vi "3 Balls.vi"() -> ()   [LabVIEW 2019]
uses:
  Team Code/TurretMode.ctl
  Team Code/MotorsGlobal.vi
  Team Code/JoysticksGlobal.vi
  Default3BallEnum.ctl
panel:
  in  "TimeLimit_Atira":dbl
  in  "3BallPID":enum32{"AndaAtras1", "AlinhaLL"}(tab)
  in  "DistanceAtras1":dbl
  in  "DelayAndaAtras1":i32=300
  in  "TimeLimit_AlinhaLL":dbl
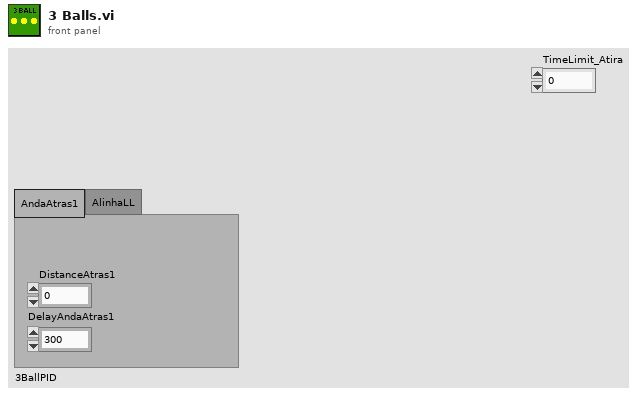
[diagram p1: front panel]
types:
  T1 = typedef "TurretMode.ctl" = enum16{"Static", "Manual", "Automatic"}
  T2 = typedef "Default3BallEnum.ctl" = enum16{"Reset1", "AndaAtras1", "AlinhaLL", "Atira"}
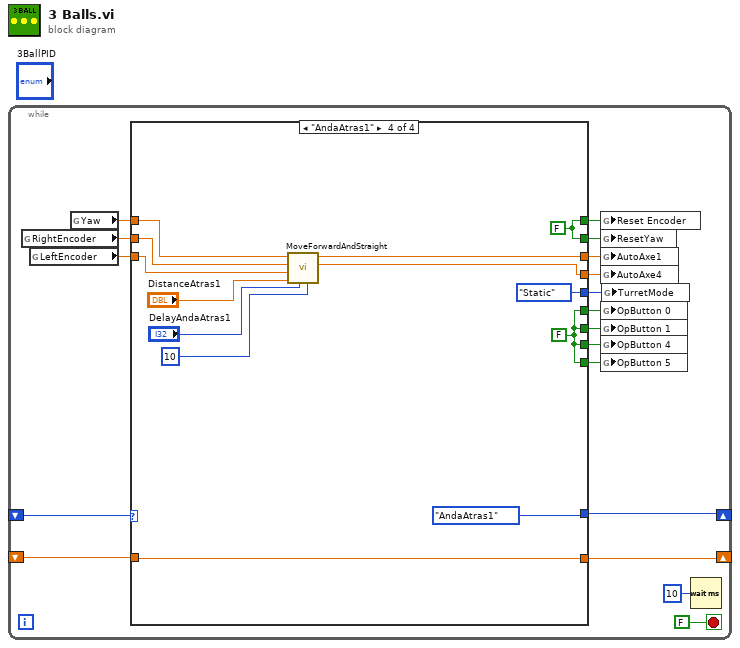
[diagram p0: block diagram]
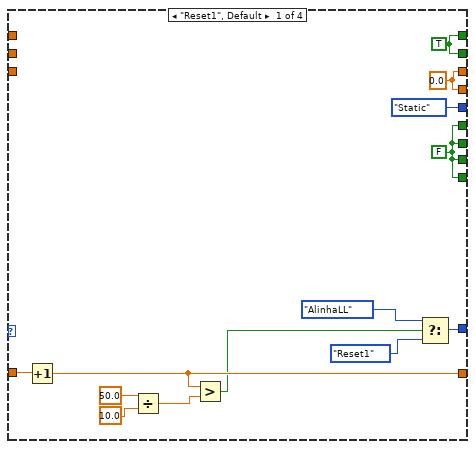
[diagram p2: hidden frame]
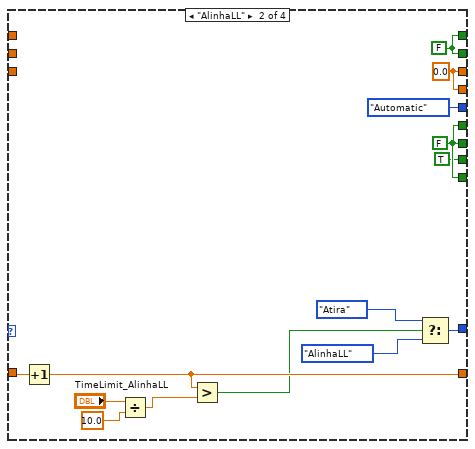
[diagram p3: hidden frame]
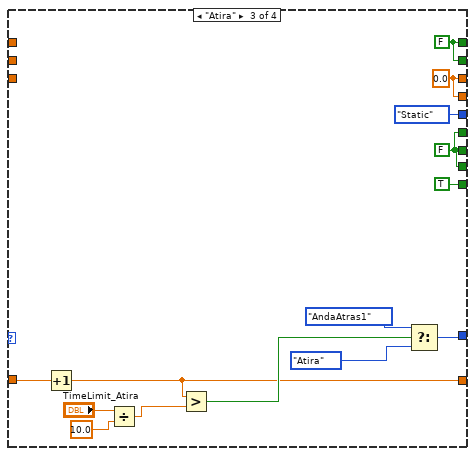
[diagram p4: hidden frame]
diagram:
  n1 = while {
    shift-right: [w15] -> _
    shift-left: _ -> [w16]
    shift-right: [w13] -> _
    shift-left: _ -> [w14]
    stop <- FALSE stop-if-true
    n2 = global read "MotorsGlobal.vi" "RightEncoder"() -> (w2:dbl)
    n3 = global read "MotorsGlobal.vi" "LeftEncoder"() -> (w1:dbl)
    n4 = global read "MotorsGlobal.vi" "Yaw"() -> (w3:dbl)
    n5 = case shown="\"AndaAtras1\"" w16 {
      tunnel: [w30 w34 w48 Default3BallEnum."AndaAtras1"] -> w15
      tunnel: w14 -> [w26 w41 w47 w61]
      tunnel: [w25 w37 w46 w61] -> w13
      tunnel: [w22 w44 w58 w63] -> w12
      tunnel: [w22 w44 w58 w63] -> w11
      tunnel: [w22 TRUE w58 w63] -> w10
      tunnel: [w22 w44 TRUE w63] -> w9
      tunnel: [w21 w45 w56 w64] -> w8
      tunnel: [w21 w45 w56 w64] -> w7
      tunnel: [TurretMode."Static" ("TurretMode") TurretMode."Automatic" ("TurretMode") TurretMode."Static" ("TurretMode") TurretMode."Static" ("TurretMode")] -> w6
      tunnel: [w19 w42 w57 w69] -> w5
      tunnel: [w19 w42 w57 w68] -> w4
      tunnel: w3 -> [_ _ _ w72]
      tunnel: w2 -> [_ _ _ w71]
      tunnel: w1 -> [_ _ _ w70]
      frame "Reset1", Default {
        w19 = 0.0
        w21 = TRUE
        w22 = FALSE
        n6 = Increment(x=w26) -> (x+1=w25:dbl)
        n7 = Divide(x=50.0, y=10.0) -> (x/y=w27:dbl)
        n8 = Greater?(x=w25, y=w27) -> (0:w24:bool)
        n9 = Select(t=Default3BallEnum."AlinhaLL", s=w24, f=Default3BallEnum."Reset1") -> (s? t:f=w30:T2)
      }
      frame "AlinhaLL" {
        w42 = 0.0 ("Trottle")
        w44 = FALSE
        w45 = FALSE
        n10 = Increment(x=w41) -> (x+1=w37:dbl)
        n11 = Divide(x="TimeLimit_AlinhaLL", y=10.0) -> (x/y=w38:dbl)
        n12 = Greater?(x=w37, y=w38) -> (0:w33:bool)
        n13 = Select(t=Default3BallEnum."Atira", s=w33, f=Default3BallEnum."AlinhaLL") -> (s? t:f=w34:T2)
      }
      frame "Atira" {
        w56 = FALSE
        w57 = 0.0 ("Trottle")
        w58 = FALSE
        n14 = Increment(x=w47) -> (x+1=w46:dbl)
        n15 = Divide(x="TimeLimit_Atira", y=10.0) -> (x/y=w52:dbl)
        n16 = Greater?(x=w46, y=w52) -> (0:w49:bool)
        n17 = Select(t=Default3BallEnum."AndaAtras1", s=w49, f=Default3BallEnum."Atira") -> (s? t:f=w48:T2)
      }
      frame "AndaAtras1" {
        w63 = FALSE
        w64 = FALSE
        n18 = call "MoveForwardAndStraight.vi"("Loop Timer"=10, "Time to stop"="DelayAndaAtras1", "Distance"="DistanceAtras1", "Encoder Left"=w70, "Encoder Right"=w71, "Yaw"=w72) -> ("Direction"=w68:dbl, "Trottle"=w69:dbl)  [unwired: 2 in, 2 out]
      }
    }
    n19 = global write "MotorsGlobal.vi" "Reset Encoder"(w8) -> ()
    n20 = global write "MotorsGlobal.vi" "ResetYaw"(w7) -> ()
    n21 = global write "JoysticksGlobal.vi" "AutoAxe1"(w5) -> ()
    n22 = global write "JoysticksGlobal.vi" "AutoAxe4"(w4) -> ()
    n23 = global write "JoysticksGlobal.vi" "OpButton 0"(w12) -> ()
    n24 = global write "JoysticksGlobal.vi" "OpButton 1"(w11) -> ()
    n25 = global write "JoysticksGlobal.vi" "OpButton 4"(w10) -> ()
    n26 = global write "JoysticksGlobal.vi" "OpButton 5"(w9) -> ()
    n27 = global write "MotorsGlobal.vi" "TurretMode"(w6) -> ()
    n28 = Wait (ms)(milliseconds to wait=u32 10) -> ()  [unwired: 1 out]
  }
